vi "ABB Instruments report.vi"(10 "Report in":string) -> (2 "Report out":string)   [LabVIEW 2017]
uses:
  ABB global.vi
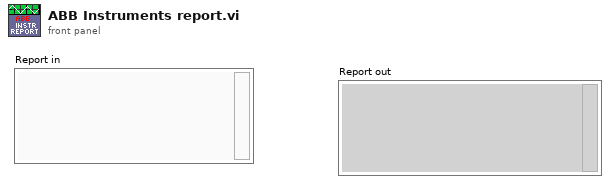
[diagram p1: front panel]
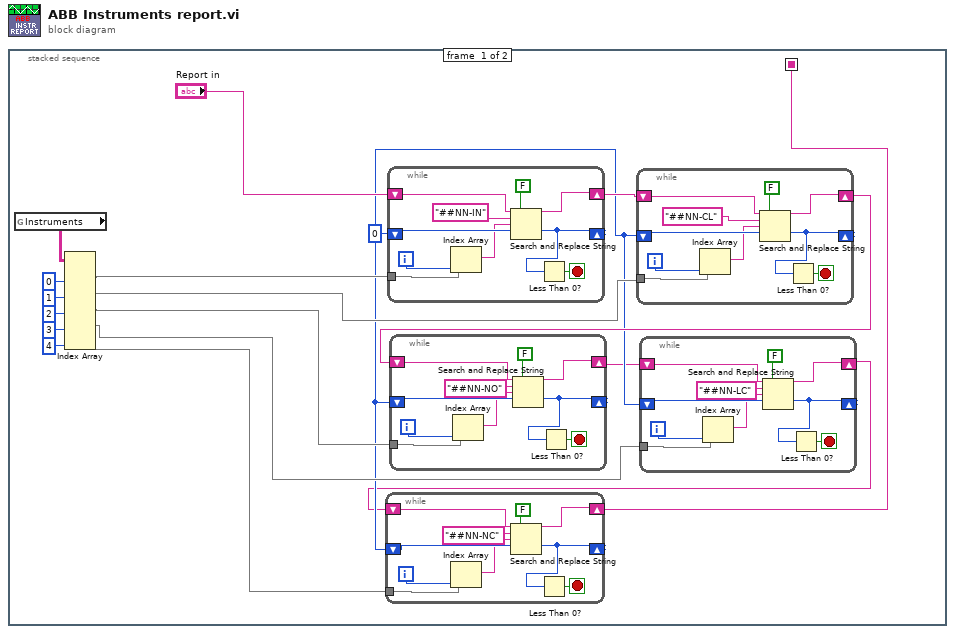
[diagram p0: block diagram]
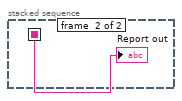
[diagram p2: hidden frame]
diagram:
  n1 = stacked-sequence {
    seq-local: [w3 _] -> [_ w69]
    frame #0 {
      w5 = 0
      n2 = global read "ABB global.vi" "Instruments"() -> (w16:string[][])
      n3 = Index Array(array=w16, index (col) #1=0 ("disabled index (col)"), index (col) #2=1 ("index (col)"), index (col) #3=2 ("index (col)"), index (col) #4=3 ("index (col)"), index (col) #5=4 ("index (col)")) -> (element #1=w10:string[], element #2=w9:string[], element #3=w7:string[], element #4=w6:string[], element #5=w4:string[])  [unwired: 5 in]
      n4 = while {
        shift-right: [w66] -> w17
        shift-left: "Report in" -> [w68]
        tunnel: w10 -> [w61]
        shift-right: [w62] -> _
        shift-left: w5 -> [w65]
        i -> [w60]
        stop <- w63 stop-if-true
        n5 = Index Array(array=w61, index=w60) -> (element=w59:string)
        n6 = Search and Replace String(replace all?=FALSE ("replace all? (F)"), input string=w68, search string="##NN-IN", replace string=w59, offset=w65) -> (result string=w66:string, offset past replacement=w62:i32)  [unwired: 3 in, 2 out]
        n7 = Less Than 0?(x=w62) -> (x < 0?=w63:bool)
      }
      n8 = while {
        shift-right: [w56] -> w8
        shift-left: w17 -> [w58]
        tunnel: w9 -> [w51]
        shift-right: [w52] -> _
        shift-left: w5 -> [w55]
        i -> [w50]
        stop <- w53 stop-if-true
        n9 = Index Array(array=w51, index=w50) -> (element=w49:string)
        n10 = Search and Replace String(replace all?=FALSE ("replace all? (F)"), input string=w58, search string="##NN-CL", replace string=w49, offset=w55) -> (result string=w56:string, offset past replacement=w52:i32)  [unwired: 3 in, 2 out]
        n11 = Less Than 0?(x=w52) -> (x < 0?=w53:bool)
      }
      n12 = while {
        shift-right: [w46] -> w1
        shift-left: w8 -> [w48]
        tunnel: w7 -> [w41]
        shift-right: [w42] -> _
        shift-left: w5 -> [w45]
        i -> [w40]
        stop <- w43 stop-if-true
        n13 = Index Array(array=w41, index=w40) -> (element=w39:string)
        n14 = Search and Replace String(replace all?=FALSE ("replace all? (F)"), input string=w48, search string="##NN-NO", replace string=w39, offset=w45) -> (result string=w46:string, offset past replacement=w42:i32)  [unwired: 3 in, 2 out]
        n15 = Less Than 0?(x=w42) -> (x < 0?=w43:bool)
      }
      n16 = while {
        shift-right: [w36] -> w2
        shift-left: w1 -> [w38]
        tunnel: w6 -> [w31]
        shift-right: [w32] -> _
        shift-left: w5 -> [w35]
        i -> [w30]
        stop <- w33 stop-if-true
        n17 = Index Array(array=w31, index=w30) -> (element=w29:string)
        n18 = Search and Replace String(replace all?=FALSE ("replace all? (F)"), input string=w38, search string="##NN-LC", replace string=w29, offset=w35) -> (result string=w36:string, offset past replacement=w32:i32)  [unwired: 3 in, 2 out]
        n19 = Less Than 0?(x=w32) -> (x < 0?=w33:bool)
      }
      n20 = while {
        shift-right: [w26] -> w3
        shift-left: w2 -> [w28]
        tunnel: w4 -> [w21]
        shift-right: [w22] -> _
        shift-left: w5 -> [w25]
        i -> [w20]
        stop <- w23 stop-if-true
        n21 = Index Array(array=w21, index=w20) -> (element=w19:string)
        n22 = Search and Replace String(replace all?=FALSE ("replace all? (F)"), input string=w28, search string="##NN-NC", replace string=w19, offset=w25) -> (result string=w26:string, offset past replacement=w22:i32)  [unwired: 3 in, 2 out]
        n23 = Less Than 0?(x=w22) -> (x < 0?=w23:bool)
      }
    }
    frame #1 {
      "Report out" <- w69
    }
  }
